vi "dual daq connection.vi"() -> ()   [LabVIEW 2025]
uses:
  <vilib>/DAQmx/read.llb/DAQmx Read (Analog 1D Wfm NChan NSamp).vi
  <vilib>/DAQmx/create/channels.llb/DAQmx Create Channel (AI-Temperature-Thermocouple).vi
  <vilib>/DAQmx/configure/timing.llb/DAQmx Timing (Sample Clock).vi
  <vilib>/DAQmx/miscellaneous.llb/DAQmx Fill In Error Info.vi
  <vilib>/Utility/file.llb/Write Delimited Spreadsheet (DBL).vi
panel:
  in  "physical channels":tag
  out "elapse time":dbl
  in  "?":bool
  in  "Seconds":dbl
  out "Waveform Graph":dbl[][](graph)
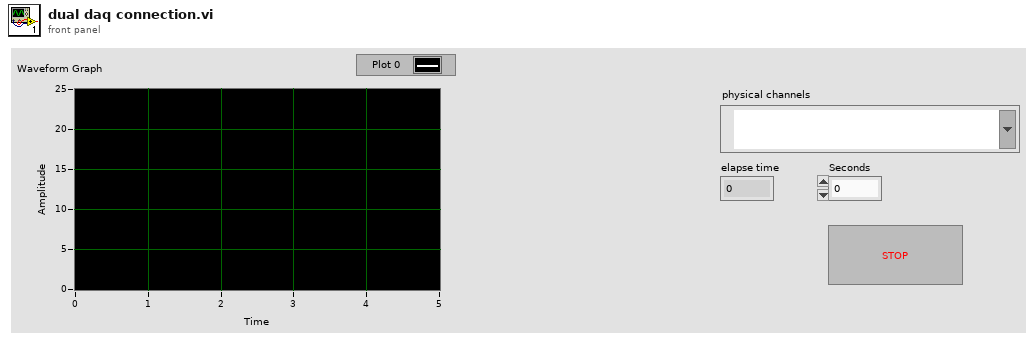
[diagram p1: front panel]
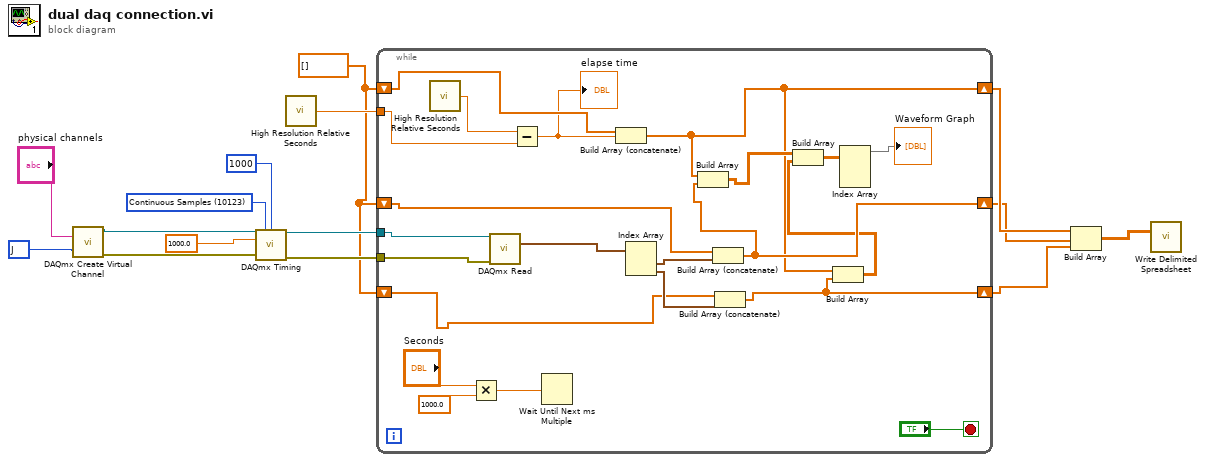
[diagram p0: block diagram]
diagram:
  w5 = dbl[] []
  w12 = 10123 items=["Finite Samples"=10178, "Continuous Samples"=10123, "Hardware Timed Single Point"=12522] ("sample mode")
  w15 = 10072 items=["J"=10072, "K"=10073, "N"=10077, "R"=10082, "S"=10085, "T"=10086, "B"=10047, "E"=10055, "A"=16208, "C"=16209] ("thermocouple type")
  n1 = call-poly <vilib>:"DAQmx Create Virtual Channel.vi"("physical channels"="physical channels", "thermocouple type"=w15) -> ("task out"=w14:refnum<k21>, "error out"=w13:errorcluster)  [unwired: 12 in]
  n2 = call-poly <vilib>:"DAQmx Timing.vi"("task/channels in"=w14, "sample mode"=w12, "samples per channel"=1000, "rate"=1000.0, "error in"=w13) -> ("task out"=w10:refnum<k21>, "error out"=w9:errorcluster)  [unwired: 9 in]
  n3 = call <vilib>:"High Resolution Relative Seconds.vi"() -> ("relative seconds"=w8:dbl)
  n4 = while {
    tunnel: w10 -> [w37]
    tunnel: w9 -> [w36]
    shift-right: [w22] -> w3
    shift-left: w5 -> [w33]
    shift-right: [w19] -> w2
    shift-left: w5 -> [w31]
    tunnel: w8 -> [w25]
    shift-right: [w20] -> w4
    shift-left: w5 -> [w24]
    stop <- "?" stop-if-true
    n5 = call <vilib>:"High Resolution Relative Seconds.vi"() -> ("relative seconds"=w26:dbl)
    n6 = Multiply(x="Seconds", y=1000.0) -> (x*y=w30:dbl)
    n7 = call-poly <vilib>:"DAQmx Read.vi"("task/channels in"=w37, "error in"=w36) -> ("data"=w35:waveform(dbl)[])  [unwired: 11 in, 2 out]
    n8 = Subtract(x=w26, y=w25) -> (x-y=w23:dbl)
    "elapse time" <- w23
    n9 = Wait Until Next ms Multiple(millisecond multiple=w30) -> ()  [unwired: 1 out]
    n10 = Build Array (concatenate)(w24, w23) -> (w20:dbl[])
    n11 = Index Array(array=w35) -> (element #1=w34:waveform(dbl), element #2=w32:waveform(dbl))  [unwired: 2 in]
    n12 = Build Array (concatenate)(w33, w34) -> (w22:dbl[])
    n13 = Build Array(w20, w22) -> (w21:dbl[][])
    n14 = Build Array (concatenate)(w31, w32) -> (w19:dbl[])
    n15 = Build Array(w20, w19) -> (w18:dbl[][])
    n16 = Build Array(w21, w18) -> (w17:dbl[][][])
    n17 = Index Array(array=w17) -> (element=→"Waveform Graph":dbl[][])  [unwired: 3 in]
  }
  n18 = Build Array(w4, w3, w2) -> (w1:dbl[][])
  n19 = call-poly <vilib>:"Write Delimited Spreadsheet.vi"("2D data"=w1) -> ()  [unwired: 13 in, 2 out]
